vi "SMU Switch Handshaking - LV code improvements - Streaming3.vi"(8 "error in":errorcluster, 10 "gRPCid":T1, 11 "file path (use dialog)":path=path "C:/Users/IES/Desktop/jsontestfile.json") -> (0 "error out":errorcluster, 3 "Elapsed Time":u32)   [LabVIEW 2019]
uses:
  labview-grpc-query-server/VIs/MeasurementServer_gRPCid.ctl
  <instrlib>/niDCPower/nidcpower.llb/niDCPower Send Software Edge Trigger - Signal.ctl
  labview-grpc-query-server/VIs/MeasurementServer_FourProbeRawData.ctl
  labview-grpc-query-server/VIs/MeasurementServer_ErrorOutData.ctl
  <instrlib>/niDCPower/nidcpower.llb/niDCPower Configure Software Edge Start Trigger.vi
  <instrlib>/niDCPower/nidcpower.llb/niDCPower Configure Software Edge Sequence Advance Trigger.vi
  labview-grpc-query-server/VIs/labview-grpc-measurement-server.lvlib
  SupportVIs.lvlib
panel:
  out "Numeric":i32
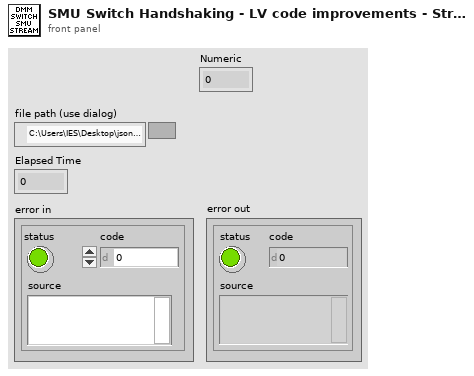
[diagram p1: front panel]
types:
  T1 = typedef "labview-grpc-measurement-server.lvlib/MeasurementServer_gRPCid.ctl" = u64
  T2 = typedef "niDCPower Send Software Edge Trigger - Signal.ctl" = i32
  T3 = typedef "JSONCluster.ctl" = cluster{"SMUResourceName":string, "SMUChannels":string, "SMUSourceMode_Sequence":i32, "SMUOutputFunction_DCCurrent":i32, "SMUSourceTransientResponse_Fast":i32, "SMUCurrent":dbl, "SMUCurrentLevelRange":dbl, "SMUMeasurementSense_Local":i32, "SMUMeasurementApertureTime":dbl, "SMUSourceAdvancedSourceDelay":dbl, "SMUVoltage":dbl, "SMUSourceAdvancedSequenceLoopCount":i32, "SMUMeasurementAdvancedDCNoiseRejection_Normal":i32, "SMUSequenceName":string, "SMUStep1_Source_DCCurrent_CurrentLevel":i32, "SMUStep2_Measurement_ApertureTime":i32, "SMUStep3_Source_Advanced_SourceDelay":i32, "SMUSequenceNumberOfSteps":i32, "SMUTriggerFromSwitch_StartDigitalEdge":string, "SMUTriggerFromSwitch_SequenceAdvanceDigitalEdge":string, "SMUTriggerToDMM_SourceCompleteEvent":i32, "SMUTriggerToDMM_SourceCompleteEvent_Value":string, "SMUTriggerToSwitch_SequenceIterationCompleteEvent":i32, "SMUTriggerToDMM_SequenceIterationCompleteEvent_Value":string, "Switch1ResourceName":string, "Switch1Topology":string, "Switch1ScanList":string, "Switch2ResourceName":string, "Switch2Topology":string, "Switch2ScanList":string, "DMMResourceName":string, "DMMFunction_DCVolts":i32, "DMMResolution":dbl, "DMMRange":dbl, "DMMTriggerSource_TTL2":i32, "DMMTriggerSlope_RisingEdge":i32, "DMMSampleTrigger_TTL2":i32, "DMMSampleCount":i32, "DMMSampleTriggerSlope_RisingEdge":i32, "DMMApertureTimeUnits_Seconds":i32, "DMMApertureTime":dbl, "DMMNumberOfAverages":i32, "DMMAutoZero_Off":i32, "DMMADCCalibration_Off":i32, "DMMSettleTime":dbl, "DMMControlAction_Commit":i32, "ApplicationNumberOfWeldChannels":i32}
  T4 = typedef "labview-grpc-measurement-server.lvlib/MeasurementServer_ErrorOutData.ctl" = cluster{"ErrorCode":i32, "ErrorMessage":string}
  T5 = typedef "labview-grpc-measurement-server.lvlib/MeasurementServer_FourProbeRawData.ctl" = cluster{"Positive Voltage":sgl, "Positive Current":sgl, "Negative Voltage":sgl, "Negative Current":sgl, "Impedance":sgl, "ErrorOutData":T4}
  T6 = typedef "niDMM Acquisition State.ctl" = enum16{"Running", "Finished with Backlog", "Finished with no Backlog", "Paused", "No acquisition in progress"}
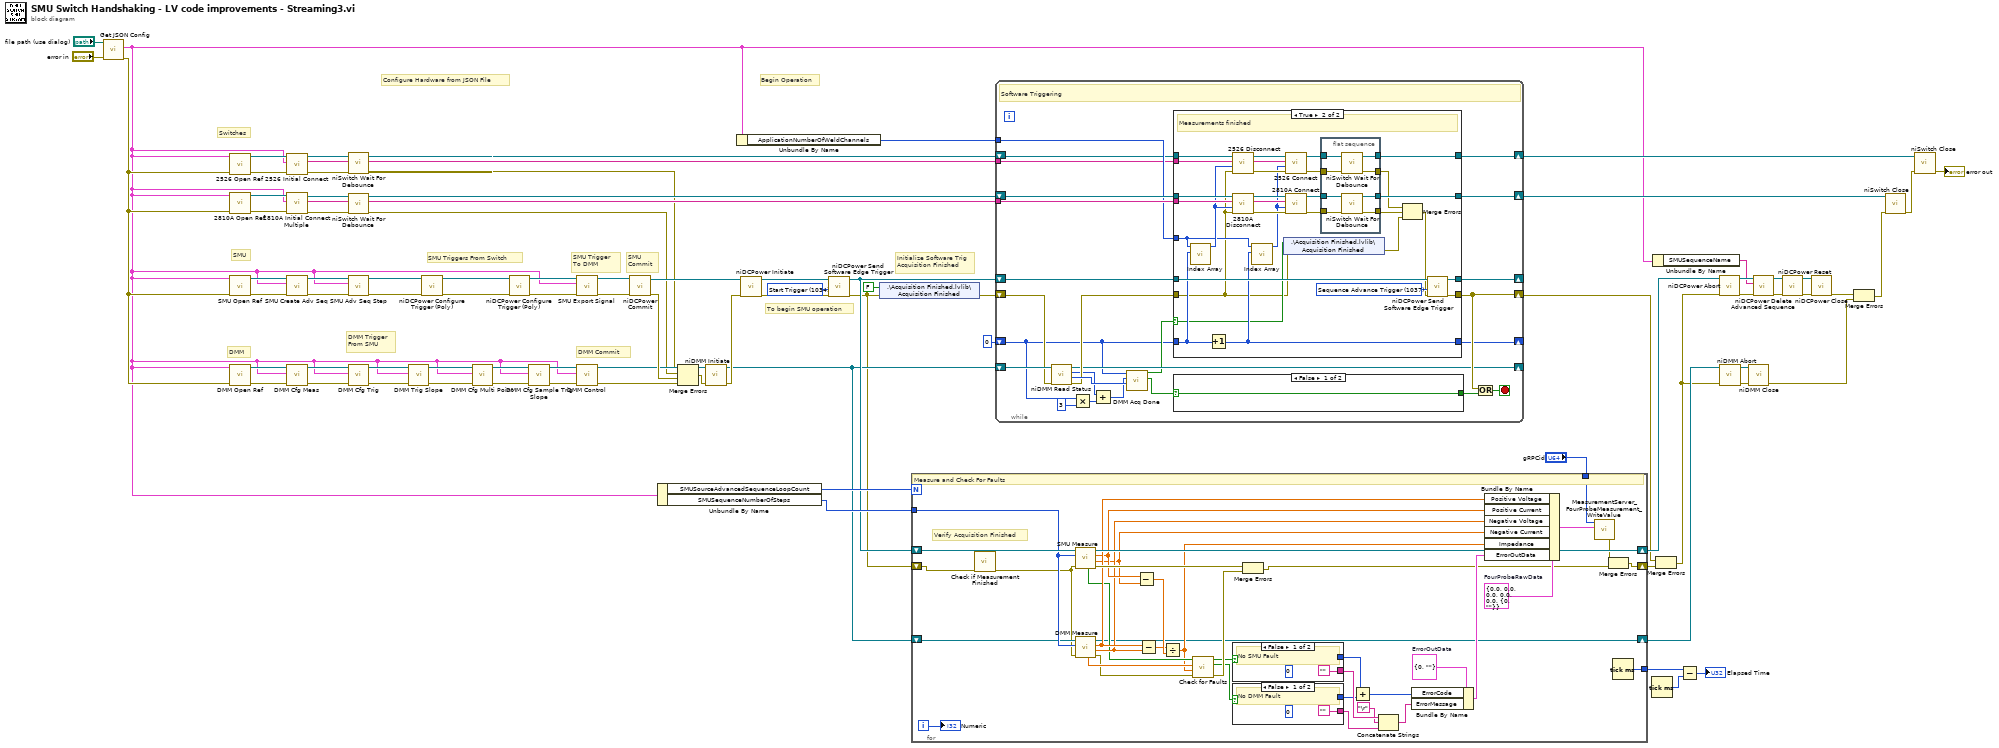
[diagram p0: block diagram]
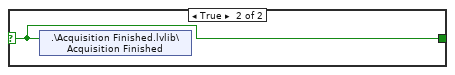
[diagram p2: hidden frame]
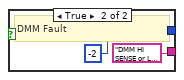
[diagram p4: hidden frame]
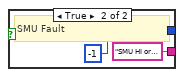
[diagram p5: hidden frame]
diagram:
  w37 = T2 1034 items=["Start Trigger"=1034, "Source Trigger"=1035, "Measure Trigger"=1036, "Sequence Advance Trigger"=1037, "Pulse Trigger"=1053] ("signal")
  # "Initialize Software Trig\nAcquisition Finished"
  # "SMU\nCommit"
  # "DMM Commit"
  # "Begin Operation"
  # "Configure Hardware from JSON File"
  # "DMM"
  # "SMU"
  # "Switches"
  # "To begin SMU operation"
  # "DMM Trigger\nFrom SMU"
  # "SMU Trigger \nTo DMM"
  # "SMU Triggers From Switch"
  n1 = call "Get JSON Config.vi"("error in (no error)"="error in", "JSON Configuration File (.json)"="file path (use dialog)") -> ("error out"=w11:errorcluster, "JSONCluster"=w5:T3)  [unwired: 6 in, 2 out]
  n2 = call "2526 Open Ref.vi"("error in"=w11, "JSONCluster"=w5) -> ("error out"=w23:errorcluster, "IVI Refnum out"=w24:refnum<k15>)  [unwired: 8 in]
  n3 = call "2810A Open Ref.vi"("error in"=w11, "JSONCluster"=w5) -> ("error out"=w30:errorcluster, "IVI Refnum out"=w31:refnum<k15>)  [unwired: 8 in]
  n4 = call "SMU Open Ref.vi"("error in (no error)"=w11, "JSONCluster"=w5) -> ("error out"=w84:errorcluster, "IVI Refnum out"=w85:refnum<k15>)  [unwired: 8 in]
  n5 = call "DMM Open Ref.vi"("error in"=w11, "JSONCluster"=w5) -> ("error out"=w57:errorcluster, "IVI Refnum out"=w56:refnum<k15>)  [unwired: 8 in]
  n6 = call "2526 Initial Connect.vi"("error in (no error)"=w23, "JSONCluster"=w5, "IVI Refnum in"=w24) -> ("error out"=w21:errorcluster, "2525 Scan List Channels"=w17:string[], "IVI Refnum out"=w22:refnum<k15>)  [unwired: 6 in]
  n7 = call "2810A Initial Connect Multiple.vi"("error in (no error)"=w30, "JSONCluster"=w5, "IVI Refnum in"=w31) -> ("error out"=w27:errorcluster, "Array"=w29:string[], "IVI Refnum out"=w28:refnum<k15>)  [unwired: 6 in]
  n8 = call "SMU Create Adv Seq.vi"("error in (no error)"=w84, "JSONCluster"=w5, "IVI Refnum in"=w85) -> ("error out"=w72:errorcluster, "IVI Refnum out"=w73:refnum<k15>)  [unwired: 7 in]
  n9 = call "DMM Cfg Meas.vi"("error in (no error)"=w57, "JSONCluster"=w5, "IVI Refnum in"=w56) -> ("error out"=w61:errorcluster, "IVI Refnum out"=w60:refnum<k15>)  [unwired: 7 in]
  n10 = call <instrlib>:"niSwitch Wait For Debounce.vi"("error in (no error)"=w21, "instrument handle"=w22) -> ("error out"=w19:errorcluster, "instrument handle out"=w18:refnum<k15>)  [unwired: 8 in]
  n11 = call <instrlib>:"niSwitch Wait For Debounce.vi"("error in (no error)"=w27, "instrument handle"=w28) -> ("error out"=w26:errorcluster, "instrument handle out"=w25:refnum<k15>)  [unwired: 8 in]
  n12 = call "SMU Adv Seq Step.vi"("error in (no error)"=w72, "JSONCluster"=w5, "IVI Refnum in"=w73) -> ("error out"=w70:errorcluster, "IVI Refnum out"=w71:refnum<k15>)  [unwired: 7 in]
  n13 = call "DMM Cfg Trig.vi"("error in (no error)"=w61, "JSONCluster"=w5, "IVI Refnum in"=w60) -> ("error out"=w63:errorcluster, "IVI Refnum out"=w62:refnum<k15>)  [unwired: 7 in]
  n14 = call "DMM Trig Slope.vi"("error in (no error)"=w63, "JSONCluster"=w5, "IVI Refnum in"=w62) -> ("error out"=w65:errorcluster, "IVI Refnum out"=w64:refnum<k15>)  [unwired: 7 in]
  n15 = call-poly <instrlib>:"niDCPower Configure Trigger (Poly).vi"("error in (no error)"=w70, "instrument handle"=w71) -> ("error out"=w81:errorcluster, "instrument handle out"=w82:refnum<k15>)  [unwired: 8 in]
  n16 = call "DMM Cfg Multi Point.vi"("error in (no error)"=w65, "JSONCluster"=w5, "IVI Refnum in"=w64) -> ("error out"=w67:errorcluster, "IVI Refnum out"=w66:refnum<k15>)  [unwired: 7 in]
  n17 = call-poly <instrlib>:"niDCPower Configure Trigger (Poly).vi"("error in (no error)"=w81, "instrument handle"=w82) -> ("error out"=w44:errorcluster, "instrument handle out"=w45:refnum<k15>)  [unwired: 8 in]
  n18 = call "DMM Cfg Sample Trig Slope.vi"("error in (no error)"=w67, "JSONCluster"=w5, "IVI Refnum in"=w66) -> ("error out"=w49:errorcluster, "IVI Refnum out"=w50:refnum<k15>)  [unwired: 7 in]
  n19 = call "SMU Export Signal.vi"("error in (no error)"=w44, "JSONCluster"=w5, "IVI Refnum in"=w45) -> ("error out"=w68:errorcluster, "IVI Refnum out"=w69:refnum<k15>)  [unwired: 7 in]
  n20 = call "DMM Control.vi"("error in (no error)"=w49, "JSONCluster"=w5, "IVI Refnum in"=w50) -> ("error out"=w54:errorcluster, "IVI Refnum out"=w51:refnum<k15>)  [unwired: 7 in]
  n21 = call <instrlib>:"niDCPower Commit.vi"("error in (no error)"=w68, "instrument handle"=w69) -> ("error out"=w55:errorcluster, "instrument handle out"=w52:refnum<k15>)  [unwired: 8 in]
  n22 = Unbundle By Name(w5) -> ("SMUSourceAdvancedSequenceLoopCount"=w40:i32, "SMUSequenceNumberOfSteps"=w39:i32)
  n23 = Merge Errors(w19, w26, w55, w54) -> (w53:errorcluster)
  n24 = call <instrlib>:"niDMM Initiate.vi"("error in (no error)"=w53, "instrument handle"=w51) -> ("error out"=w20:errorcluster, "instrument handle out"=w6:refnum<k15>)  [unwired: 8 in]
  n25 = Unbundle By Name(w5) -> ("ApplicationNumberOfWeldChannels"=w33:i32)
  n26 = call <instrlib>:"niDCPower Initiate.vi"("error in (no error)"=w20, "instrument handle"=w52) -> ("error out"=w32:errorcluster, "instrument handle out"=w38:refnum<k15>)  [unwired: 8 in]
  n27 = call <instrlib>:"niDCPower Send Software Edge Trigger.vi"("error in (no error)"=w32, "signal"=w37, "instrument handle"=w38) -> ("error out"=w3:errorcluster, "instrument handle out"=w7:refnum<k15>)  [unwired: 7 in]
  n28 = shared-variable ".\\Acquisition Finished.lvlib\\Acquisition Finished"(FALSE ("Measurement Finished"), error in=w3) -> (error out=w2:errorcluster)
  n29 = for {
    N: w40 -> [_]
    tunnel: w39 -> [w95]
    shift-right: [w93] -> w9
    shift-left: w3 -> [w87]
    shift-right: [w123] -> w83
    shift-left: w7 -> [w96]
    shift-right: [w90] -> w46
    shift-left: w6 -> [w92]
    tunnel: [w100] -> w12
    tunnel: "gRPCid" -> [w99]
    i -> [w86]
    w101 = T4 {"ErrorCode"=0, "ErrorMessage"=""}  # ErrorOutData
    w98 = T5 {"Positive Voltage"=0.0, "Positive Current"=0.0, "Negative Voltage"=0.0, "Negative Current"=0.0, "Impedance"=0.0, "ErrorOutData"={"ErrorCode"=0, "ErrorMessage"=""}}  # FourProbeRawData
    # "Verify Acquisition Finished"
    # "Measure and Check For Faults"
    n30 = call "Check if Measurement Finished"("error in (no error)"=w87) -> ("error out"=w88:errorcluster)  [unwired: 10 in]
    n31 = call "SMU Measure.vi"("error in (no error)"=w88, "SMUSequenceNumberOfSteps"=w95, "IVI Refnum in"=w96) -> ("error out"=w122:errorcluster, "Numeric"=w115:dbl, "Numeric 2"=w117:dbl, "IVI Refnum out"=w123:refnum<k15>, "in compliance"=w104:bool[])  [unwired: 4 in]
    n32 = call "DMM Measure.vi"("error in (no error)"=w88, "SMUSequenceNumberOfSteps"=w95, "IVI Refnum in"=w92) -> ("error out"=w91:errorcluster, "Numeric"=w116:dbl, "Numeric 2"=w118:dbl, "IVI Refnum out"=w90:refnum<k15>, "Measurements"=w103:dbl[])  [unwired: 4 in]
    n33 = Subtract(x=w117, y=w115) -> (x-y=w120:dbl)
    n34 = Subtract(x=w118, y=w116) -> (x-y=w119:dbl)
    n35 = Divide(x=w119, y=w120) -> (x/y=w102:dbl)
    n36 = call "Check for Faults.vi"("Error In"=w91, "Resistance In"=w102, "dmm voltage measurements"=w103, "in compliance"=w104) -> ("Error Out"=w121:errorcluster, "DMM Fault"=w108:bool, "SMU Fault"=w112:bool)  [unwired: 4 in, 1 out]
    n37 = case shown="False" w112 {
      tunnel: ["" "SMU HI or LO lead disconnected\n- SMU in compliance\n- SMU Fault = True"] -> w111
      tunnel: [0 -1] -> w109
      frame False {
        # "No SMU Fault"
      }
      frame True {
        # "SMU Fault"
      }
    }
    n38 = case shown="False" w108 {
      tunnel: ["" "DMM HI SENSE or LO SENSE lead disconnected\n- DMM measures NaN, or \n- DMM overrange warning, or\n- DMM voltage > 50uV "] -> w106
      tunnel: [0 -2] -> w105
      frame False {
        # "No DMM Fault"
      }
      frame True {
        # "DMM Fault"
      }
    }
    n39 = Merge Errors(w122, w121) -> (w89:errorcluster)
    n40 = Add(x=w109, y=w105) -> (x+y=w113:i32)
    n41 = Concatenate Strings(w111, "\r", w106) -> (w110:string)
    n42 = Bundle By Name(cluster=w101, "ErrorCode"=w113, "ErrorMessage"=w110) -> (w114:T4)
    n43 = Bundle By Name(cluster=w98, "Positive Voltage"=w118, "Positive Current"=w117, "Negative Voltage"=w116, "Negative Current"=w115, "Impedance"=w102, "ErrorOutData"=w114) -> (w97:T5)
    n44 = call "MeasurementServer_FourProbeMeasurement_WriteValue.vi"("gRPCid"=w99, "FourProbeRawData"=w97) -> ("error out"=w94:errorcluster)  [unwired: 8 in]
    n45 = Merge Errors(w94, w89) -> (w93:errorcluster)
    n46 = Tick Count (ms)() -> (millisecond timer value=w100:u32)
    "Numeric" <- w86
  }
  n47 = while {
    shift-right: [w156] -> _
    shift-left: w7 -> [w151]
    shift-right: [w154] -> w4
    shift-left: w2 -> [w139]
    shift-right: [w152] -> w34
    shift-left: w25 -> [w153]
    shift-right: [w141] -> _
    shift-left: w6 -> [w143]
    shift-right: [w150] -> _
    shift-left: 0 ("Backlog") -> [w136]
    tunnel: w29 -> [w149]
    tunnel: w33 -> [w148]
    shift-right: [w146] -> w16
    shift-left: w18 -> [w147]
    tunnel: w17 -> [w145]
    stop <- w155 stop-if-true
    # "Software Triggering"
    n48 = call <instrlib>:"niDMM Read Status.vi"("error in (no error)"=w139, "instrument handle"=w143) -> ("error out"=w142:errorcluster, "Acquisition State"=w144:T6, "Backlog"=w138:i32, "instrument handle out"=w141:refnum<k15>)  [unwired: 6 in]
    n49 = Multiply(x=w136, y=3) -> (x*y=w134:i32)
    n50 = Add(x=w138, y=w134) -> (x+y=w137:i32)
    n51 = call "DMM Acq Done.vi"("Acquisition State"=w144, "Backlog"=w137, "Channel Index"=w136) -> ("Finished with Backlog?"=w133:bool, "Sequence Acquision Finished?"=w140:bool)  [unwired: 7 in]
    n52 = case shown="True" w140 {
      selector: w140 -> [_ w166]
      tunnel: w142 -> [w162 w165]
      tunnel: [w163 w192] -> w156
      tunnel: [w162 w191] -> w154
      tunnel: w151 -> [w163 w188]
      tunnel: w153 -> [w161 w187]
      tunnel: [w161 w190] -> w152
      tunnel: w136 -> [w160 w171]
      tunnel: [w160 w168] -> w150
      tunnel: w149 -> [_ w184]
      tunnel: w148 -> [_ w167]
      tunnel: w147 -> [w159 w179]
      tunnel: [w159 w176] -> w146
      tunnel: w145 -> [_ w175]
      frame False {
        # "Measurements not finished yet - repeat loop"
      }
      frame True {
        w189 = T2 1037 items=["Start Trigger"=1034, "Source Trigger"=1035, "Measure Trigger"=1036, "Sequence Advance Trigger"=1037, "Pulse Trigger"=1053] ("signal")
        # "Measurements finished"
        n53 = call "Index Array.vi"("Backlog"=w171, "ApplicationNumberOfWeldChannels"=w167) -> ("Index"=w170:i32)  [unwired: 9 in]
        n54 = Increment(x=w171) -> (x+1=w168:i32)
        n55 = call "2526 Disconnect.vi"("error in (no error)"=w165, "Index"=w170, "2525 Scan List Channels"=w175, "IVI Refnum in"=w179) -> ("error out"=w180:errorcluster, "IVI Refnum out"=w181:refnum<k15>)  [unwired: 6 in]
        n56 = call "2810A Disconnect.vi"("error in (no error)"=w165, "Numeric"=w170, "Array"=w184, "IVI Refnum in"=w187) -> ("error out"=w183:errorcluster, "IVI Refnum out"=w186:refnum<k15>)  [unwired: 6 in]
        n57 = call "Index Array.vi"("Backlog"=w168, "ApplicationNumberOfWeldChannels"=w167) -> ("Index"=w169:i32)  [unwired: 9 in]
        n58 = shared-variable ".\\Acquisition Finished.lvlib\\Acquisition Finished"(w166, error in=w165) -> (error out=w164:errorcluster)
        n59 = call "2526 Connect.vi"("error in (no error)"=w180, "Index"=w169, "2525 Scan List Channels"=w175, "IVI Refnum in"=w181) -> ("error out"=w177:errorcluster, "IVI Refnum out"=w178:refnum<k15>)  [unwired: 6 in]
        n60 = call "2810A Connect.vi"("error in (no error)"=w183, "Index"=w169, "Array"=w184, "IVI Refnum in"=w186) -> ("error out"=w182:errorcluster, "IVI Refnum out"=w185:refnum<k15>)  [unwired: 6 in]
        n61 = flat-sequence {
          tunnel: [w200] -> w190
          tunnel: [w199] -> w174
          tunnel: w185 -> [w198]
          tunnel: w182 -> [w197]
          tunnel: w178 -> [w196]
          tunnel: w177 -> [w195]
          tunnel: [w194] -> w176
          tunnel: [w193] -> w173
          frame #0 {
            n62 = call <instrlib>:"niSwitch Wait For Debounce.vi"("error in (no error)"=w195, "instrument handle"=w196) -> ("error out"=w193:errorcluster, "instrument handle out"=w194:refnum<k15>)  [unwired: 8 in]
            n63 = call <instrlib>:"niSwitch Wait For Debounce.vi"("error in (no error)"=w197, "instrument handle"=w198) -> ("error out"=w199:errorcluster, "instrument handle out"=w200:refnum<k15>)  [unwired: 8 in]
          }
        }
        n64 = Merge Errors(w173, w174, w164) -> (w172:errorcluster)
        n65 = call <instrlib>:"niDCPower Send Software Edge Trigger.vi"("error in (no error)"=w172, "signal"=w189, "instrument handle"=w188) -> ("error out"=w191:errorcluster, "instrument handle out"=w192:refnum<k15>)  [unwired: 7 in]
      }
    }
    n66 = case shown="False" w133 {
      selector: w133 -> [w157 w158]
      tunnel: [w157 w158] -> w132
      frame False {
      }
      frame True {
        n67 = shared-variable ".\\Acquisition Finished.lvlib\\Acquisition Finished"(w158) -> ()  [unwired: 1 in, 1 out]
      }
    }
    n68 = Or(x=w154, y=w132) -> (x .or. y?=w155:bool)
  }
  n69 = Tick Count (ms)() -> (millisecond timer value=w80:u32)
  n70 = Unbundle By Name(w5) -> ("SMUSequenceName"=w13:string)
  n71 = Merge Errors(w4, w9) -> (w8:errorcluster)
  n72 = Subtract(x=w12, y=w80) -> (x-y=→"Elapsed Time":u32)
  n73 = call <instrlib>:"niDCPower Abort.vi"("error in (no error)"=w8, "instrument handle"=w83) -> ("error out"=w78:errorcluster, "instrument handle out"=w79:refnum<k15>)  [unwired: 8 in]
  n74 = call <instrlib>:"niDMM Abort.vi"("error in (no error)"=w8, "instrument handle"=w46) -> ("error out"=w59:errorcluster, "instrument handle out"=w58:refnum<k15>)  [unwired: 8 in]
  n75 = call <instrlib>:"niDMM Close.vi"("error in (no error)"=w59, "instrument handle"=w58) -> ("error out"=w48:errorcluster)  [unwired: 9 in]
  n76 = call <instrlib>:"niDCPower Delete Advanced Sequence.vi"("error in (no error)"=w78, "sequence name"=w13, "instrument handle"=w79) -> ("error out"=w77:errorcluster, "instrument handle out"=w76:refnum<k15>)  [unwired: 7 in]
  n77 = call <instrlib>:"niDCPower Reset.vi"("error in (no error)"=w77, "instrument handle"=w76) -> ("error out"=w74:errorcluster, "instrument handle out"=w75:refnum<k15>)  [unwired: 2 in, 6 out]
  n78 = call <instrlib>:"niDCPower Close.vi"("error in (no error)"=w74, "instrument handle"=w75) -> ("error out"=w47:errorcluster)  [unwired: 9 in]
  n79 = Merge Errors(w47, w48) -> (w35:errorcluster)
  n80 = call <instrlib>:"niSwitch Close.vi"("error in (no error)"=w35, "instrument handle"=w34) -> ("error out"=w15:errorcluster)  [unwired: 9 out]
  n81 = call <instrlib>:"niSwitch Close.vi"("error in (no error)"=w15, "instrument handle"=w16) -> ("error out"=→"error out":errorcluster)  [unwired: 9 out]
